vi "Write Color Pixel Array.vi"(8 "error in (no error)":errorcluster, 10 "Color Pixel Array":u8[](array[numeric]), 11 "Kinect Session in":refnum<class "Kinect Session.lvclass">) -> (0 "error out":errorcluster, 3 "Kinect Session out":refnum<class "Kinect Session.lvclass">)   [LabVIEW 2014, in "Kinect Library.lvlib" / "Kinect Session.lvclass"]
uses:
  Kinect Session.lvclass
  Kinect Session.lvclass/Kinect Session.ctl
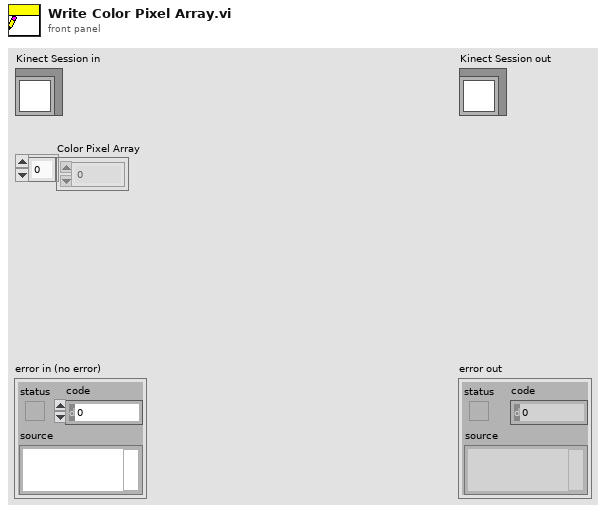
[diagram p1: front panel]
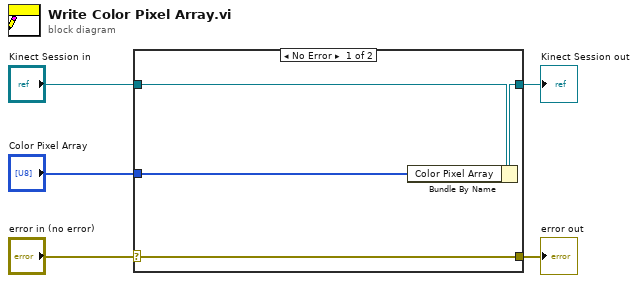
[diagram p0: block diagram]
diagram:
  n1 = case shown="No Error" "error in (no error)" {
    selector: "error in (no error)" -> [w9 w10]
    tunnel: [w9 w10] -> w4
    tunnel: [w7 w11] -> w2
    tunnel: "Kinect Session in" -> [w8 w11]
    tunnel: "Color Pixel Array" -> [w6 _]
    frame No Error {
      n2 = Bundle By Name(cluster=w8, "Color Pixel Array"=w6) -> (w7:refnum<class "Kinect Session.lvclass">)
    }
    frame Error {
    }
  }
  "error out" <- w4
  "Kinect Session out" <- w2
